vi "Get User Interface Information.vi"(8 "error in (no error)":errorcluster, 11 "Continuous Counting Mesurement2 in":refnum<class "Continuous Counting Measurement2.lvclass">) -> (0 "error out":errorcluster, 2 "user interface information":T1[](array[typedef]), 3 "Continuous Counting Mesurement2 out":refnum<class "Continuous Counting Measurement2.lvclass">)   [LabVIEW 2021, in "MeasurementServerTests.lvlib" / "Measurement Service Tests.lvlib" / "Continuous Counting Measurement2.lvclass"]
doc: "Provides information about the user interfaces supported by the measurement if any. The user interface file can be specified using either a relative or absolute paths. When using a relative path, the path should be relative to the Measurement Logic.vi for the measurement."
uses:
  Continuous Counting Measurement2.lvclass
  Runtime/Measurements/Helpers/TypeDefs/User Interface Information.ctl
  Runtime/Measurements/NI Measurement Plug-In SDK.lvlib
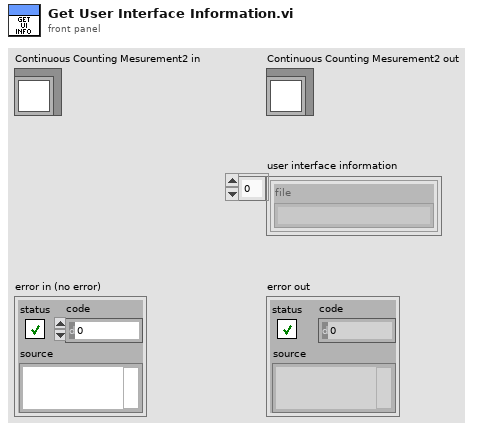
[diagram p1: front panel]
types:
  T1 = typedef "NI Measurement Plug-In SDK.lvlib/User Interface Information.ctl" = cluster{"file":string}
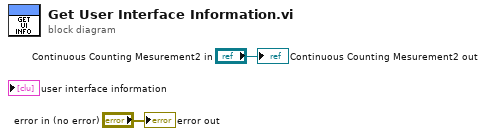
[diagram p0: block diagram]
diagram:
  "error out" <- "error in (no error)"
  "Continuous Counting Mesurement2 out" <- "Continuous Counting Mesurement2 in"
